vi "Limit Crossover Check.vi"(2 "NewVal":cluster{dbl, dbl, dbl, dbl}, 3 "OldVal":cluster{dbl, dbl, dbl, dbl}) -> (0 "Value":dbl, 1 "Index":i32)   [LabVIEW 2013]
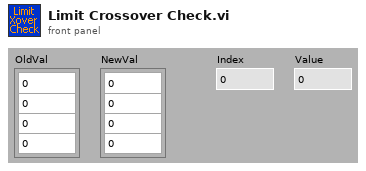
[diagram p1: front panel]
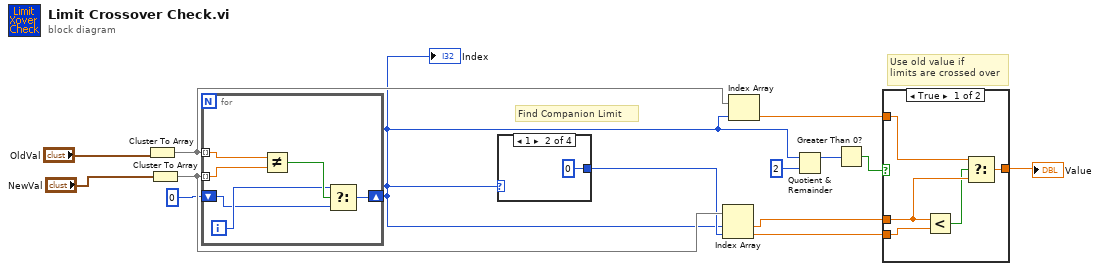
[diagram p0: block diagram]
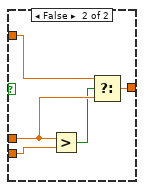
[diagram p2: hidden frame]
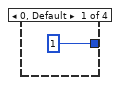
[diagram p3: hidden frame]
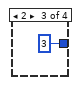
[diagram p4: hidden frame]
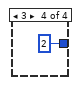
[diagram p5: hidden frame]
diagram:
  # "Use old value if\nlimits are crossed over"
  # "Find Companion Limit"
  n1 = Cluster To Array(cluster="OldVal") -> (array=w9:dbl[])
  n2 = Cluster To Array(cluster="NewVal") -> (array=w14:dbl[])
  n3 = for {
    tunnel: w9 -> [w20] mode=indexing
    shift-right: [w18] -> w2
    shift-left: 0 -> [w15]
    tunnel: w14 -> [w19] mode=indexing
    i -> [w16]
    n4 = Not Equal?(x=w20, y=w19) -> (x != y?=w17:bool)
    n5 = Select(t=w16, s=w17, f=w15) -> (s? t:f=w18:i32)
  }
  "Index" <- w2
  n6 = case shown="1" w2 {
    tunnel: [1 0 3 2] -> w10
    frame 0, Default {
    }
    frame 1 {
    }
    frame 2 {
    }
    frame 3 {
    }
  }
  n7 = Index Array(array=w14, index #1=w2, index #2=w10) -> (element #1=w5:dbl, element #2=w4:dbl)
  n8 = Index Array(array=w9, index=w2) -> (element=w3:dbl)
  n9 = Quotient & Remainder(x=w2, y=2) -> (x-y*floor(x/y)=w7:i32)  [unwired: 1 out]
  n10 = Greater Than 0?(x=w7) -> (x > 0?=w6:bool)
  n11 = case shown="True" w6 {
    tunnel: w5 -> [w28 w33]
    tunnel: w4 -> [w29 w34]
    tunnel: w3 -> [w26 w31]
    tunnel: [w25 w30] -> w1
    frame True {
      n12 = Less?(x=w28, y=w29) -> (x < y?=w27:bool)
      n13 = Select(t=w26, s=w27, f=w28) -> (s? t:f=w25:dbl)
    }
    frame False {
      n14 = Greater?(x=w33, y=w34) -> (0:w32:bool)
      n15 = Select(t=w31, s=w32, f=w33) -> (s? t:f=w30:dbl)
    }
  }
  "Value" <- w1
